vi "MSGR_Main.vi"() -> ()   [LabVIEW 2018]
uses:
  MSGR Q Name TypeDef.ctl
panel:
  out "error":errorcluster
  in  "stop":bool
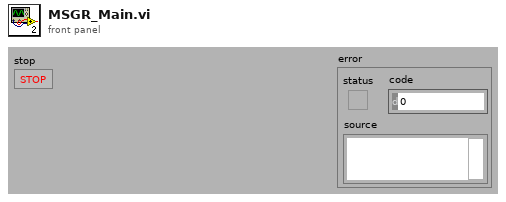
[diagram p1: front panel]
types:
  T1 = typedef "MSGR Q Name TypeDef.ctl" = string
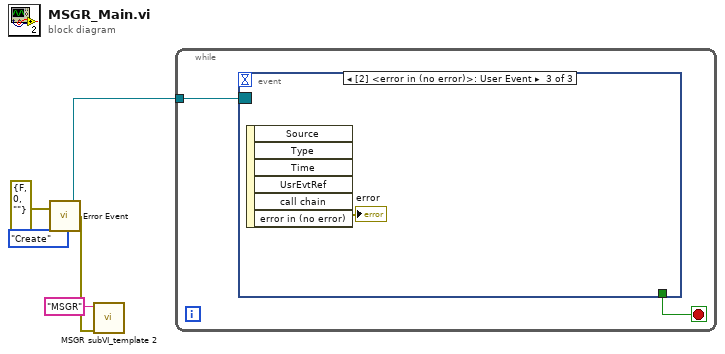
[diagram p0: block diagram]
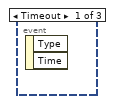
[diagram p2: hidden frame]
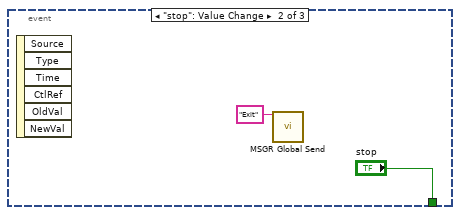
[diagram p3: hidden frame]
diagram:
  n1 = call "Error Event.vi"("error in (no error)"=errorcluster {"status"=FALSE, "code"=0, "source"=""}, "Enum"=enum16{"Create", "Default", "Destroy"}."Create") -> ("Event Registration Refnum"=w4:refnum<event-registration>, "error out"=w2:errorcluster)  [unwired: 4 in]
  n2 = call "MSGR subVI_template 2.vi"("error in (no error)"=w2, "MSGR Q name"=T1 "MSGR") -> ()  [unwired: 9 in, 1 out]
  n3 = while {
    tunnel: w4 -> [w7]
    stop <- w6 stop-if-true
    n4 = event shown="[2] <error in (no error)>: User Event" {
      selector: w7 -> [_ _ _]
      dyn-events: _ -> [_ _ _]
      timeout: _ -> [_ _ _]
      tunnel: [_ "stop" _] -> w6
      event Timeout {
        n5 = event-data() -> ()  [unwired: 3 out]
      }
      event "stop": Value Change {
        n6 = event-data() -> ()  [unwired: 7 out]
        n7 = call "MSGR Global Send.vi"("Msg"="Exit") -> ()  [unwired: 5 in, 10 out]
      }
      event User Event {
        n8 = event-data() -> ("error in (no error)"=→"error":errorcluster)  [unwired: 6 out]
      }
    }
  }
